vi "Yokogawa GS200 VSweep.vi"(0 "UP Limit (V)":dbl=10.0 min=-32.0 max=32.0 format="%.5f", 1 "GPIB Address":refnum<visa-resource-name>="GPIB0::11::INSTR", 3 "Step Size (mV)":dbl=100.0 format="%.4f", 4 "Sweep":bool=TRUE, 5 "HOLD UL":bool, 6 "Initial V":dbl format="%.6f", 9 "LW Limit (V)":dbl=-10.0 min=-32.0 max=32.0 format="%.5f", 10 "Goto (V)":dbl format="%.6f", 11 "HOLD LL":bool, 12 "Sweep Rate UP (mV/s)":dbl=100.0 format="%.3f", 14 "Sweep Rate DN (mV/s)":dbl=100.0 format="%.3f", 15 "stop":bool) -> (8 "Boolean":bool)   [LabVIEW 2025]
doc: "Author: Scott Hannahs <sth@magnet.fsu.edu>\n\nThis software is licensed for use under the “MIT License\"\nCopyright (c) 2025 Scott Hannahs, sth@sth@magnet.sthnet.net\n\nPermission is hereby granted, free of charge, to any person obtaining a copy of this software and associated documentation files (the \"Software\"), to deal in the Software without restriction, including without limitation the rights to use, copy, modify, merge, publish, distribute, sublicense, and/or sell copies of the Software, and to permit persons to whom the Software is furnished to do so, subject to the following conditions: The above copyright notice and this permission notice shall be included in all copies or substantial portions of the Software.\n\nTHE SOFTWARE IS PROVIDED \"AS IS\", WITHOUT WARRANTY OF ANY KIND, EXPRESS OR IMPLIED, INCLUDING BUT NOT LIMITED TO THE WARRANTIES OF MERCHANTABILITY, FITNESS FOR A PARTICULAR PURPOSE AND NONINFRINGEMENT. IN NO EVENT SHALL THE AUTHORS OR COPYRIGHT HOLDERS BE LIABLE FOR ANY CLAIM, DAMAGES OR OTHER LIABILITY, WHETHER IN AN ACTION OF CONTRACT, TORT OR OTHERWISE, ARISING FROM, OUT OF OR IN CONNECTION WITH THE SOFTWARE OR THE USE OR OTHER DEALINGS IN THE SOFTWARE."
panel:
  out "Now at (V)":dbl format="%.6f"
  out "Status":enum16{"Sweep DN", "Sweep UP", "Fixed V"}(ring)
  in  "Initialize Flag":bool
  out "error out 2":T1
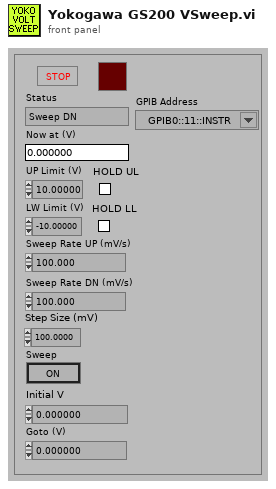
[diagram p1: front panel]
types:
  T1 = cluster{"error":bool, "code":i32, "source":string}
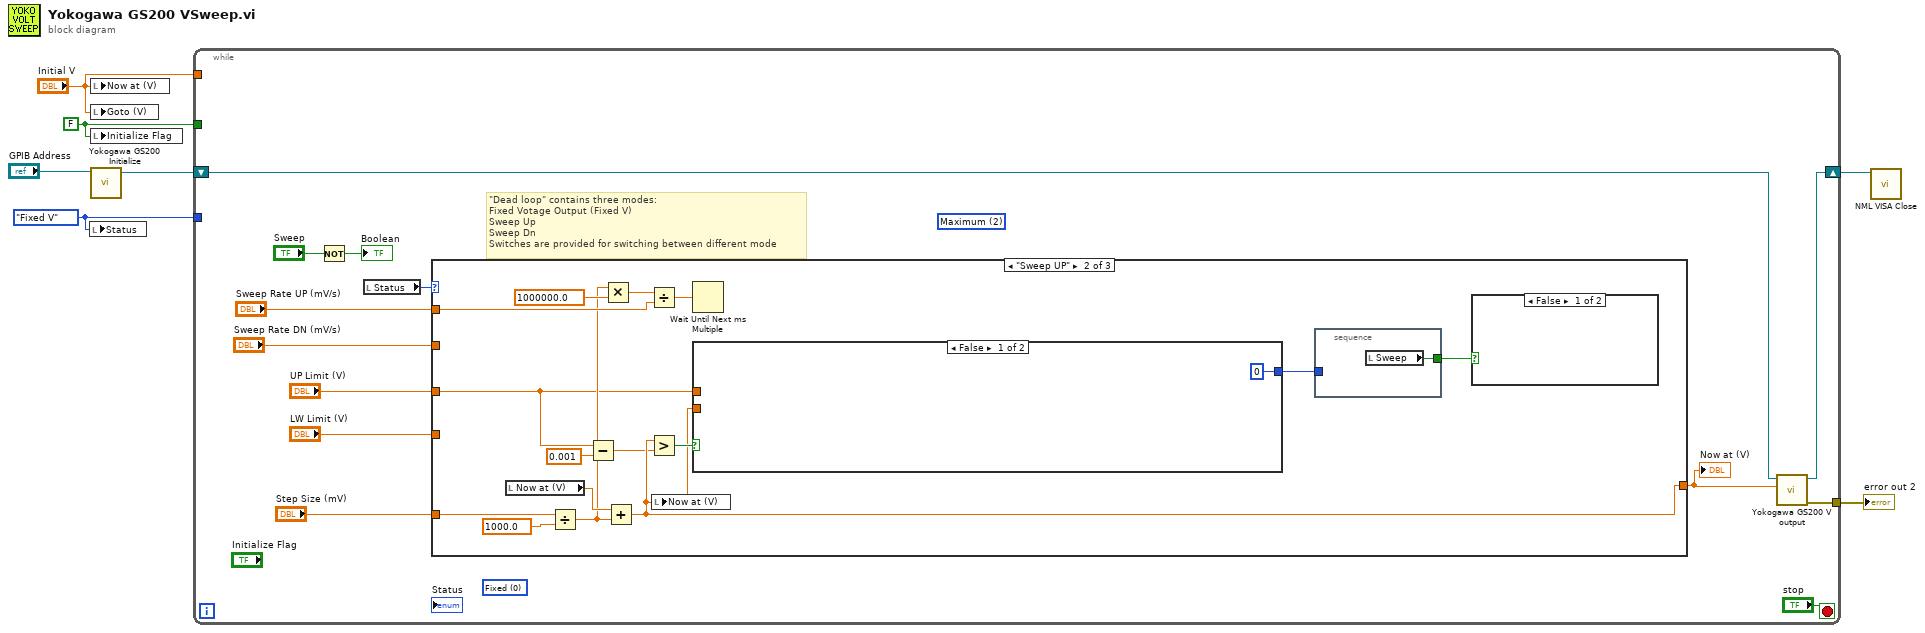
[diagram p0: block diagram]
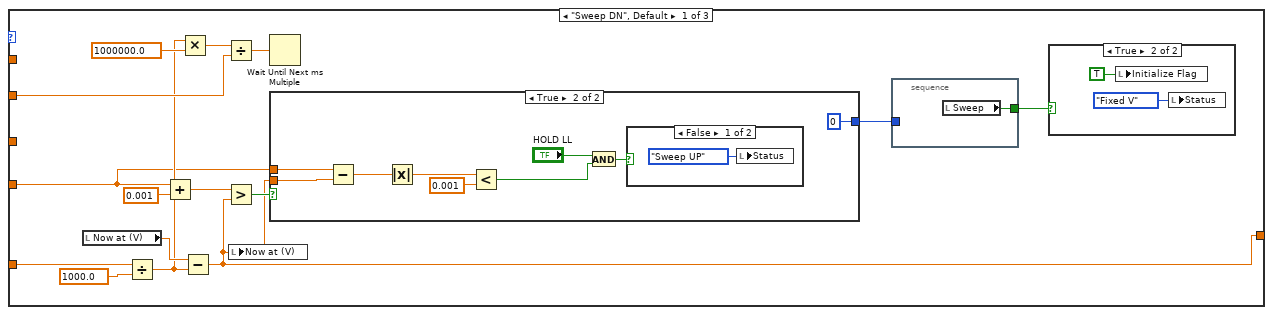
[diagram p2: hidden frame]
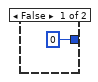
[diagram p4: hidden frame]
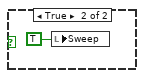
[diagram p5: hidden frame]
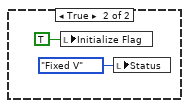
[diagram p6: hidden frame]
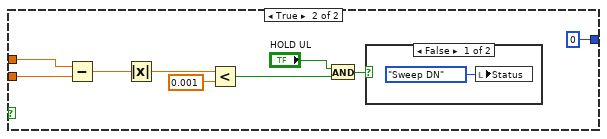
[diagram p7: hidden frame]
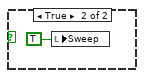
[diagram p8: hidden frame]
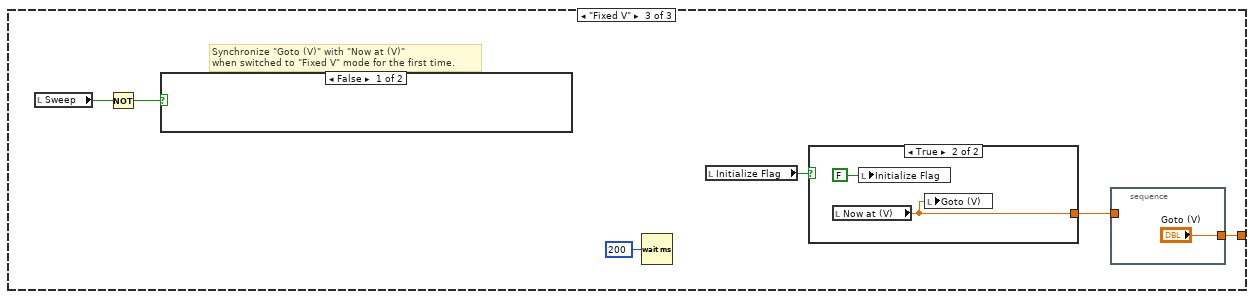
[diagram p9: hidden frame]
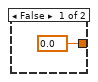
[diagram p10: hidden frame]
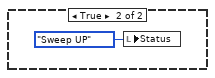
[diagram p11: hidden frame]
diagram:
  w5 = FALSE ("Initialize Flag")
  w6 = enum16{"Sweep DN", "Sweep UP", "Fixed V"}."Fixed V" ("Status")
  n1 = local write "Status"(w6) -> ()
  n2 = local write "Now at (V)"("Initial V") -> ()
  n3 = local write "Goto (V)"("Initial V") -> ()
  n4 = local write "Initialize Flag"(w5) -> ()
  n5 = call "Yokogawa GS200 Initialize.vi"("VISA resource name"="GPIB Address") -> ("dup VISA Session"=w2:refnum<visa-resource-name>)  [unwired: 3 in, 2 out]
  n6 = while {
    tunnel: [w11] -> w7
    tunnel: "Initial V" -> [_]
    tunnel: w6 -> [_]
    tunnel: w5 -> [_]
    shift-right: [w8] -> w1
    shift-left: w2 -> [w9]
    stop <- "stop" stop-if-true
    (unwired) u16 2 items=["Default 20V Range", "Minimum", "Maximum", "By Value", "Auto On", "Auto Off"] ("Range (Default:0)")
    (unwired) u16 0 items=["Fixed", "Sweep", "List"] ("Mode Selection (Fixed:0)")
    # "\"Dead loop\" contains three modes:\nFixed Votage Output (Fixed V)\nSweep Up\nSweep Dn\nSwitches are provided for switching between different mode"
    n7 = Not(x="Sweep") -> (.not. x?=→"Boolean":bool)
    n8 = local read "Status"() -> (w16:enum16{"Sweep DN", "Sweep UP", "Fixed V"})
    n9 = case shown="\"Sweep UP\"" w16 {
      tunnel: "Sweep Rate UP (mV/s)" -> [_ w61 _]
      tunnel: "UP Limit (V)" -> [_ w51 _]
      tunnel: "LW Limit (V)" -> [w21 _ _]
      tunnel: "Sweep Rate DN (mV/s)" -> [w33 _ _]
      tunnel: [w22 w54 w86] -> w10
      tunnel: "Step Size (mV)" -> [w28 w56 _]
      frame "Sweep DN", Default {
        n10 = local read "Now at (V)"() -> (w35:dbl)
        n11 = Divide(x=w28, y=1000.0) -> (x/y=w26:dbl)
        n12 = Add(x=w21, y=0.001) -> (x+y=w23:dbl)
        n13 = Multiply(x=w26, y=1000000.0) -> (x*y=w34:dbl)
        n14 = Subtract(x=w35, y=w26) -> (x-y=w22:dbl)
        n15 = Divide(x=w34, y=w33) -> (x/y=w32:dbl)
        n16 = Greater?(x=w23, y=w22) -> (0:w31:bool)
        n17 = local write "Now at (V)"(w22) -> ()
        n18 = Wait Until Next ms Multiple(millisecond multiple=w32) -> ()  [unwired: 1 out]
        n19 = case shown="True" w31 {
          tunnel: [0 0] -> w25
          tunnel: w22 -> [_ w46]
          tunnel: w21 -> [_ w47]
          frame False {
          }
          frame True {
            n20 = Subtract(x=w47, y=w46) -> (x-y=w45:dbl)
            n21 = Absolute Value(x=w45) -> (abs(x)=w44:dbl)
            n22 = Less?(x=w44, y=0.001) -> (x < y?=w40:bool)
            n23 = And(x="HOLD LL", y=w40) -> (x .and. y?=w42:bool)
            n24 = case shown="False" w42 {
              frame False {
                n25 = local write "Status"(enum16{"Sweep DN", "Sweep UP", "Fixed V"}."Sweep UP" ("Status")) -> ()
              }
              frame True {
                n26 = local write "Sweep"(TRUE ("Sweep")) -> ()
              }
            }
          }
        }
        n27 = stacked-sequence {
          tunnel: [w36] -> w30
          tunnel: w25 -> [_]
          frame #0 {
            n28 = local read "Sweep"() -> (w36:bool)
          }
        }
        n29 = case shown="True" w30 {
          frame False {
          }
          frame True {
            n30 = local write "Initialize Flag"(TRUE ("Initialize Flag")) -> ()
            n31 = local write "Status"(enum16{"Sweep DN", "Sweep UP", "Fixed V"}."Fixed V" ("Status")) -> ()
          }
        }
      }
      frame "Sweep UP" {
        n32 = local read "Now at (V)"() -> (w65:dbl)
        n33 = Divide(x=w56, y=1000.0) -> (x/y=w57:dbl)
        n34 = Subtract(x=w51, y=0.001) -> (x-y=w52:dbl)
        n35 = Multiply(x=w57, y=1000000.0) -> (x*y=w63:dbl)
        n36 = Add(x=w65, y=w57) -> (x+y=w54:dbl)
        n37 = Divide(x=w63, y=w61) -> (x/y=w64:dbl)
        n38 = Greater?(x=w54, y=w52) -> (0:w60:bool)
        n39 = local write "Now at (V)"(w54) -> ()
        n40 = Wait Until Next ms Multiple(millisecond multiple=w64) -> ()  [unwired: 1 out]
        n41 = case shown="False" w60 {
          tunnel: [0 0] -> w55
          tunnel: w51 -> [_ w77]
          tunnel: w54 -> [_ w76]
          frame False {
          }
          frame True {
            n42 = Subtract(x=w77, y=w76) -> (x-y=w73:dbl)
            n43 = Absolute Value(x=w73) -> (abs(x)=w72:dbl)
            n44 = Less?(x=w72, y=0.001) -> (x < y?=w70:bool)
            n45 = And(x="HOLD UL", y=w70) -> (x .and. y?=w75:bool)
            n46 = case shown="False" w75 {
              frame False {
                n47 = local write "Status"(enum16{"Sweep DN", "Sweep UP", "Fixed V"}."Sweep DN" ("Status")) -> ()
              }
              frame True {
                n48 = local write "Sweep"(TRUE ("Sweep")) -> ()
              }
            }
          }
        }
        n49 = stacked-sequence {
          tunnel: [w66] -> w59
          tunnel: w55 -> [_]
          frame #0 {
            n50 = local read "Sweep"() -> (w66:bool)
          }
        }
        n51 = case shown="False" w59 {
          frame False {
          }
          frame True {
            n52 = local write "Initialize Flag"(TRUE ("Initialize Flag")) -> ()
            n53 = local write "Status"(enum16{"Sweep DN", "Sweep UP", "Fixed V"}."Fixed V" ("Status")) -> ()
          }
        }
      }
      frame "Fixed V" {
        # "Synchronize \"Goto (V)\" with \"Now at (V)\"\nwhen switched to \"Fixed V\" mode for the first time."
        n54 = local read "Sweep"() -> (w83:bool)
        n55 = Not(x=w83) -> (.not. x?=w82:bool)
        n56 = case shown="False" w82 {
          frame False {
          }
          frame True {
            n57 = local write "Status"(enum16{"Sweep DN", "Sweep UP", "Fixed V"}."Sweep UP" ("Status")) -> ()
          }
        }
        n58 = Wait (ms)(milliseconds to wait=u32 200) -> ()  [unwired: 1 out]
        n59 = local read "Initialize Flag"() -> (w85:bool)
        n60 = case shown="True" w85 {
          tunnel: [0.0 ("Now at  (V)") w88] -> w84
          frame False {
          }
          frame True {
            n61 = local read "Now at (V)"() -> (w88:dbl)
            n62 = local write "Initialize Flag"(FALSE ("Initialize Flag")) -> ()
            n63 = local write "Goto (V)"(w88) -> ()
          }
        }
        n64 = stacked-sequence {
          tunnel: ["Goto (V)"] -> w86
          tunnel: w84 -> [_]
          frame #0 {
          }
        }
      }
    }
    "Now at (V)" <- w10
    n65 = call "Yokogawa GS200 V output.vi"("VISA resource name"=w9, "Voltage Level (0.0 V)"=w10) -> ("VISA resource name out"=w8:refnum<visa-resource-name>, "error out"=w11:errorcluster)  [unwired: 5 in]
  }
  "error out 2" <- w7
  n66 = call "NML VISA Close.vi"("VISA resource name"=w1) -> ()  [unwired: 10 in, 1 out]
